vi "add tag to default data table.vi"(8 "error in":errorcluster, 10 "system tag":refnum<class "tag descriptor.lvclass">, 11 "data dictionary in":refnum<class "data dictionary.lvclass">) -> (0 "error out":errorcluster, 3 "data dictionary out":refnum<class "data dictionary.lvclass">)   [LabVIEW 2013, in "tag bus.lvlib" / "data dictionary.lvclass"]
doc: "Adds a single tag to the default data table, converting the contained default value into a new element of the specified type, and appending that to the table."
uses:
  data dictionary.lvclass
  tag/tag descriptor.lvclass
  data dictionary.lvclass/data dictionary.ctl
  tag/tag descriptor.lvclass/tag descriptor.ctl
  tag/read data type.vi
  tag/read default value.vi
  tag/default value polymorphs/read default value Double.vi
  tag/default value polymorphs/read default value Single.vi
  tag/default value polymorphs/read default value I64.vi
  tag/default value polymorphs/read default value I32.vi
  tag/default value polymorphs/read default value I16.vi
  tag/default value polymorphs/read default value I8.vi
  tag/default value polymorphs/read default value U64.vi
  tag/default value polymorphs/read default value U32.vi
  tag/default value polymorphs/read default value U16.vi
  tag/default value polymorphs/read default value U8.vi
  tag/default value polymorphs/read default value String.vi
  tag/default value polymorphs/read default value Boolean.vi
  tag/default value polymorphs/read default value Array of U8.vi
  tag/default value polymorphs/read default value Array of U16.vi
  tag/default value polymorphs/read default value Array of U32.vi
  tag/default value polymorphs/read default value Array of U64.vi
  tag/default value polymorphs/read default value Array of I64.vi
  tag/default value polymorphs/read default value Array of I32.vi
  tag/default value polymorphs/read default value Array of I16.vi
  tag/default value polymorphs/read default value Array of I8.vi
  tag/default value polymorphs/read default value Array of Double.vi
  tag/default value polymorphs/read default value Array of Single.vi
  tag/default value polymorphs/read default value Array of Boolean.vi
  tag/default value polymorphs/read default value Array of String.vi
  table/data table.lvlib
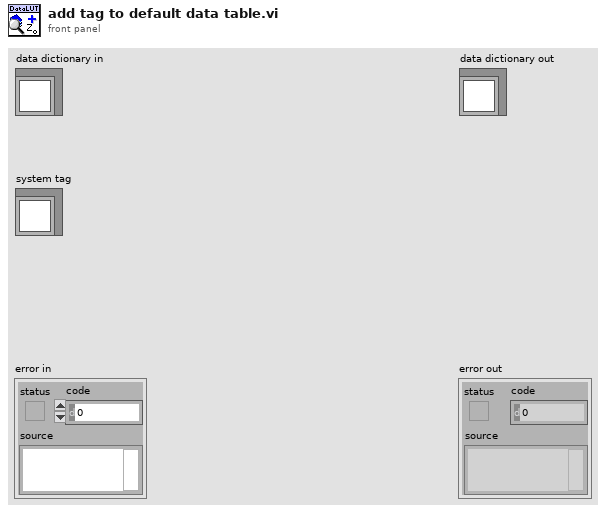
[diagram p1: front panel]
types:
  T1 = typedef "tag bus.lvlib/data table.lvlib/data table.ctl" = cluster{"Double":dbl[], "Single":sgl[], "I64":i64[], "I32":i32[], "I16":i16[], "I8":i8[], "U64":u64[], "U32":u32[], "U16":u16[], "U8":u8[], "Boolean":bool[], "String":string[], "Array of Double":cluster{"DBL Array":dbl[]}[], "Array of Single":cluster{"SGL Array":sgl[]}[], "Array of I64":cluster{"I64 Array":i64[]}[], "Array of I32":cluster{"I32 Array":i32[]}[], "Array of I16":cluster{"I16 Array":i16[]}[], "Array of I8":cluster{"I8 Array":i8[]}[], "Array of U64":cluster{"U64 Array":u64[]}[], "Array of U32":cluster{"U32 Array":u32[]}[], "Array of U16":cluster{"U16 Array":u16[]}[], "Array of U8":cluster{"U8 Array":u8[]}[], "Array of Boolean":cluster{"Boolean Array":bool[]}[], "Array of String":cluster{"String Array":string[]}[]}
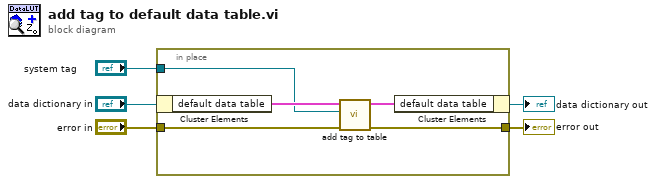
[diagram p0: block diagram]
diagram:
  n1 = in-place {
    in-place-border: "system tag" -> [w9]
    in-place-border: "error in" -> [w7]
    in-place-border: [w6] -> w1
    n2 = in-place-cluster #1("data dictionary in") -> ("default data table"=w10:T1)
    n3 = call "add tag to table.vi"("error in"=w7, "system tag"=w9, "data table in"=w10) -> ("error out"=w6:errorcluster, "data table out"=w8:T1)  [unwired: 7 in]
    n4 = in-place-cluster #1("default data table"=w8) -> (→"data dictionary out":refnum<class "data dictionary.lvclass">)
  }
  "error out" <- w1
